vi "PID.vi"() -> ()   [LabVIEW 2011]
panel:
  out "Respuestas RPM":dynamicdata(graph)=[{"t0"=timestamp(3469223810.91554 s since 1904-01-01), "dt"=1.0, "Y"=[-14.854463065672341]}, {"t0"=timestamp(3469223810.91654 s since 1904-01-01), "dt"=1.0, "Y"=[0.0]}, {"t0"=timestamp(3469223810.91654 s since 1904-01-01), "dt"=1.0, "Y"=[0.13558651620376666]}]
  out "y(k)":dbl=0.0006016765992441921
  out "RPM planta":dbl(knob)=-14.854463065672341 scale=0.0..4000.0
  out "Vo":dbl=0.0006
  in  "PID out Range":bool
  out "Senal de error":dynamicdata(graph)=[{"t0"=timestamp(3469223810.924541 s since 1904-01-01), "dt"=1.0, "Y"=[0.006363203383503446]}]
  in  "Stop":bool
  out "Senal de control (Volts)":dbl=0.09293207435418632
  out "Acciones de control PID":dynamicdata(graph)=[{"t0"=timestamp(3469223810.925541 s since 1904-01-01), "dt"=1.0, "Y"=[0.00027494100867620457]}, {"t0"=timestamp(3469223810.925541 s since 1904-01-01), "dt"=1.0, "Y"=[0.09087289111677575]}, {"t0"=timestamp(3469223810.925541 s since 1904-01-01), "dt"=1.0, "Y"=[0.001784242228734366]}, {"t0"=timestamp(3469223810.925541 s since 1904-01-01), "dt"=1.0, "Y"=[0.09293207435418632]}]
  in  "Upper Limit":dbl=5.0
  in  "Lower Limit":dbl
  out "Error RPMs":dynamicdata(graph)=[{"t0"=timestamp(3469223810.91554 s since 1904-01-01), "dt"=1.0, "Y"=[-14.854463065672341]}]
  in  "Kp":dbl=0.2804
  in  "Ki":dbl=8.0547
  in  "Kd":dbl=0.00089201
  out "Lectura LM331":dynamicdata(graph)=[{"t0"=timestamp(3469223810.924541 s since 1904-01-01), "dt"=1.0, "Y"=[-0.005763203383503446]}] caption="Lectura LM331 (Vo)"
  in  "RPM reference":dbl(slide) scale=0.0..3600.0
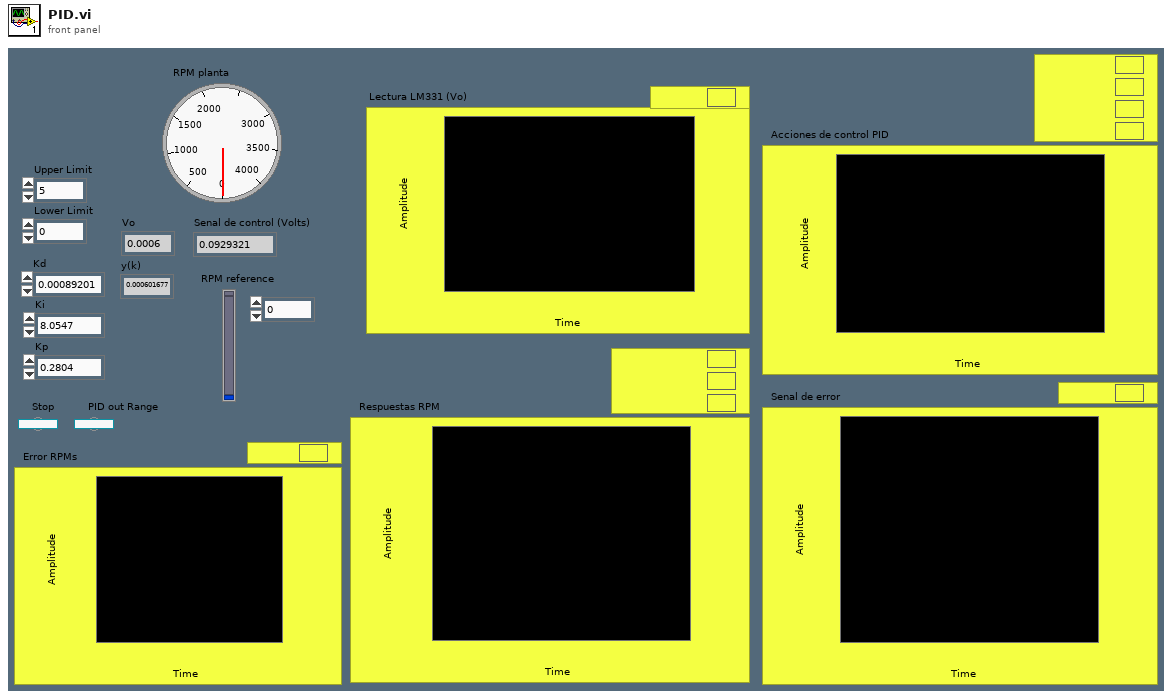
[diagram p1: front panel]
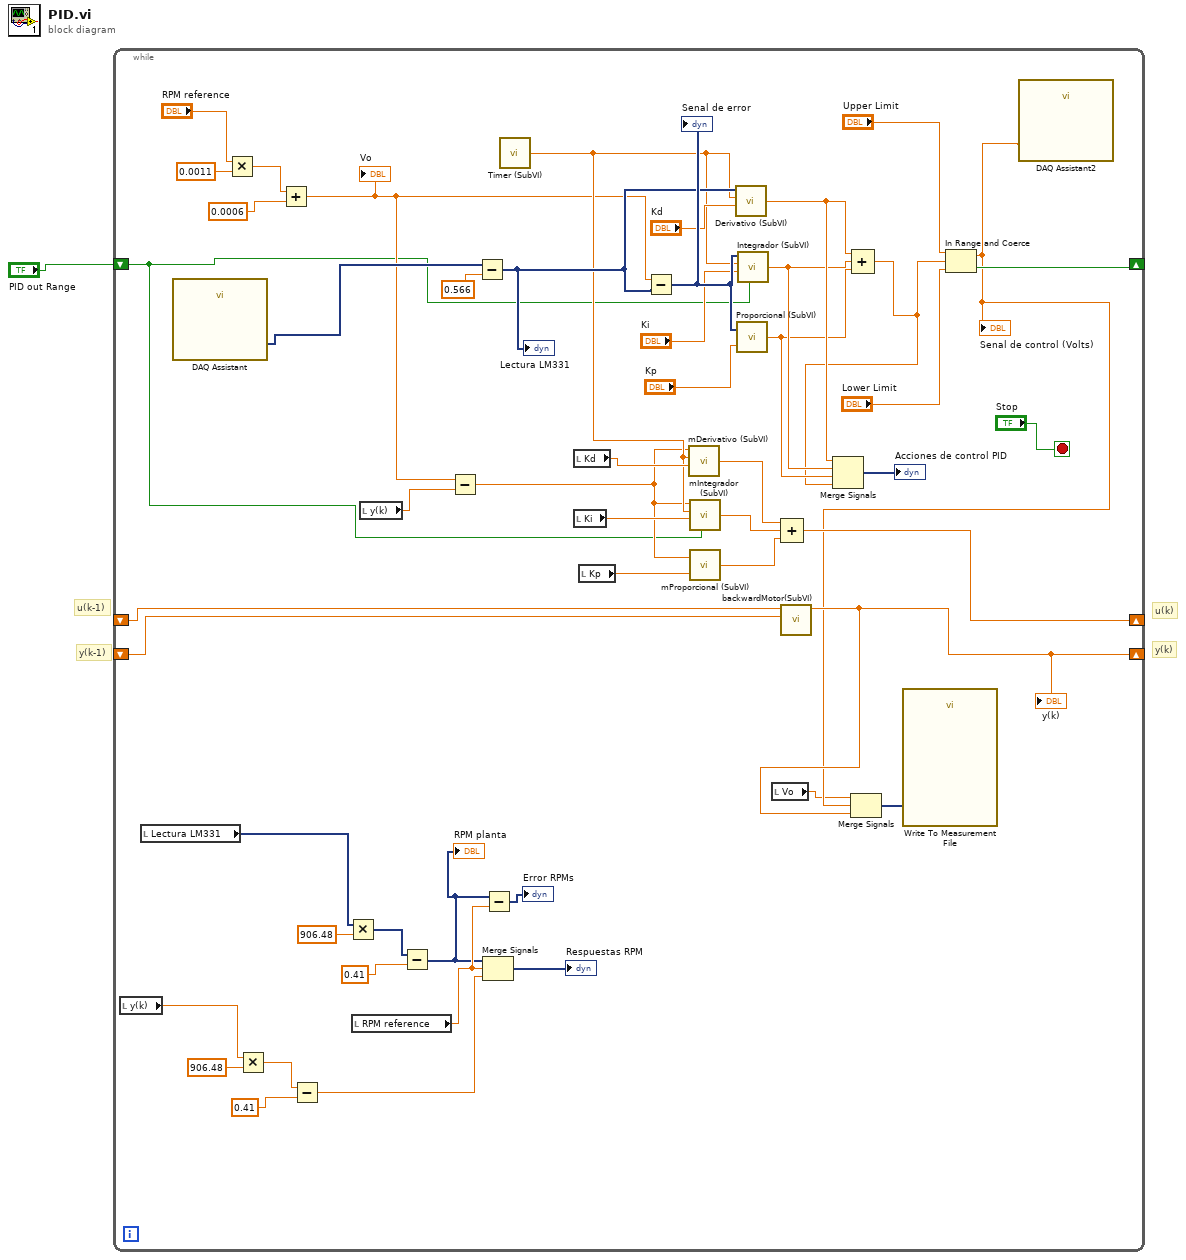
[diagram p0: block diagram]
diagram:
  # "y(k-1)"
  # "y(k)"
  # "u(k)"
  # "u(k-1)"
  n1 = while {
    shift-right: [w36] -> _
    shift-left: "PID out Range" -> [w6]
    shift-right: [w8] -> _
    shift-left: _ -> [w19]
    shift-right: [w4] -> _
    shift-left: _ -> [w20]
    stop <- "Stop" stop-if-true
    n2 = local read "y(k)"() -> (w25:dbl)
    n3 = local read "Lectura LM331"() -> (w49:dynamicdata)
    n4 = call "DAQ Assistant"() -> ("data"=w30:dynamicdata)  [unwired: 17 in, 2 out]
    n5 = Multiply(x="RPM reference", y=0.0011) -> (x*y=w47:dbl)
    n6 = Multiply(x=w25, y=906.48) -> (x*y=w27:dbl)
    n7 = Add(x=w47, y=0.0006) -> (x+y=w13:dbl)
    "Vo" <- w13
    n8 = Subtract(x=w27, y=0.41) -> (x-y=w24:dbl)
    n9 = Multiply(x=w49, y=906.48) -> (x*y=w51:dynamicdata)
    n10 = local read "RPM reference"() -> (w31:dbl)
    n11 = local read "y(k)"() -> (w12:dbl)
    n12 = Subtract(x=w51, y=0.41) -> (x-y=w29:dynamicdata)
    "RPM planta" <- w29
    n13 = Subtract(x=w13, y=w12) -> (x-y=w14:dbl)
    n14 = Subtract(x=w30, y=0.566) -> (x-y=w33:dynamicdata)
    "Lectura LM331" <- w33
    n15 = Merge Signals(w29, w31, w24) -> (→"Respuestas RPM":dynamicdata)
    n16 = Subtract(x=w29, y=w31) -> (x-y=→"Error RPMs":dynamicdata)
    n17 = call "Timer (SubVI).vi"() -> ("T"=w17:dbl)  [unwired: 1 in]
    n18 = local read "Kd"() -> (w18:dbl)
    n19 = local read "Ki"() -> (w16:dbl)
    n20 = local read "Kp"() -> (w15:dbl)
    n21 = Subtract(x=w13, y=w33) -> (x-y=w46:dynamicdata)
    "Senal de error" <- w46
    n22 = call "mDerivativo (SubVI).vi"("Kd"=w18, "T"=w17, "Vm"=w14) -> ("Accion Derivativa"=w11:dbl)  [unwired: 1 in]
    n23 = call "mIntegrador (SubVI).vi"("PID sale de rango"=w6, "Ki"=w16, "T"=w17, "Error"=w14) -> ("Accion Integral"=w10:dbl)  [unwired: 2 in]
    n24 = call "mProporcional (SubVI).vi"("Kp"=w15, "Error"=w14) -> ("Accion Proporcional"=w9:dbl)
    n25 = call "Derivativo (SubVI).vi"("Kd"="Kd", "T"=w17, "Vm"=w33) -> ("Accion Derivativa"=w40:dbl)  [unwired: 1 in]
    n26 = call "Proporcional (SubVI).vi"("Kp"="Kp", "Error"=w46) -> ("Accion Proporcional"=w38:dbl)
    n27 = call "Integrador (SubVI).vi"("PID sale de rango"=w6, "Ki"="Ki", "T"=w17, "Error"=w46) -> ("Accion Integral"=w39:dbl)  [unwired: 2 in]
    n28 = local read "Vo"() -> (w2:dbl)
    n29 = Compound Arithmetic op=ADD(w11, w10, w9) -> (w8:dbl)
    n30 = call "backwardMotor(SubVI).vi"("y(k-1)"=w20, "u(k-1)"=w19) -> ("y(k)"=w4:dbl)  [unwired: 9 in]
    "y(k)" <- w4
    n31 = Compound Arithmetic op=ADD(w40, w39, w38) -> (w7:dbl)
    n32 = Merge Signals(w40, w39, w38, w7) -> (→"Acciones de control PID":dynamicdata)
    n33 = In Range and Coerce(upper limit="Upper Limit", x=w7, lower limit="Lower Limit") -> (coerced(x)=w3:dbl, In Range?=w36:bool)
    "Senal de control (Volts)" <- w3
    n34 = Merge Signals(w2, w3, w4) -> (w5:dynamicdata)
    n35 = call "Write To Measurement File"("Signals"=w5) -> ()  [unwired: 16 in, 3 out]
    n36 = call "DAQ Assistant2"("data"=w3) -> ()  [unwired: 17 in, 2 out]
  }
